vi "FPS get.vi"() -> (0 "FPS":dbl)   [LabVIEW 2016]
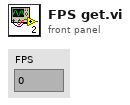
[diagram p1: front panel]
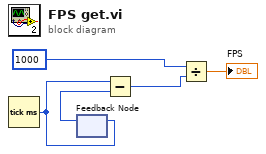
[diagram p0: block diagram]
diagram:
  n1 = Tick Count (ms)() -> (millisecond timer value=w4:u32)
  n2 = feedback #1() -> (w5:u32)  [unwired: 1 in]
  n3 = feedback-in #1(w4) -> ()
  n4 = Subtract(x=w4, y=w5) -> (x-y=w3:u32)
  n5 = Divide(x=u32 1000, y=w3) -> (x/y=→"FPS":dbl)
